vi "Log.vi"(9 "data":variant, 10 "message":string, 11 "level":T1) -> ()   [LabVIEW 2018, in "Logging.lvlib" / "Registry.lvlib"]
uses:
  Registry.lvlib
  Log Levels.ctl
  Log Action Data.ctl
  Registry Actions.ctl
  Logging.lvlib
  Utilities/Utilities.lvlib
panel:
  # "Connector Pane"
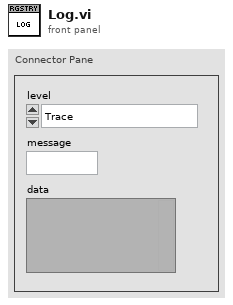
[diagram p1: front panel]
types:
  T1 = typedef "Logging.lvlib/Log Levels.ctl" = enum16{"Trace", "Debug", "Info", "Warning", "Error", "Critical"}
  T2 = typedef "Logging.lvlib/Registry.lvlib/Registry Actions.ctl" = enum16{"Register", "Log", "Enable", "Enable All", "Disable", "Disable All", "List", "Unregister", "Unregister All"}
  T3 = typedef "Logging.lvlib/Registry.lvlib/Log Action Data.ctl" = cluster{"level":T1, "message":string, "data":variant}
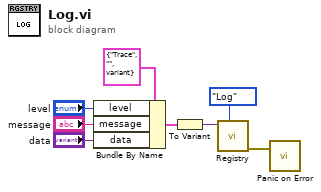
[diagram p0: block diagram]
diagram:
  n1 = Bundle By Name(cluster=T3 {"level"=enum."Trace", "message"="", "data"=variant}, "level"="level", "message"="message", "data"="data") -> (w6:T3)
  n2 = To Variant(anything=w6) -> (Variant=w7:variant)
  n3 = call "Registry.vi"("action"=Registry_Actions."Log", "data in"=w7) -> ("error out"=w1:errorcluster)  [unwired: 8 in, 1 out]
  n4 = call "Panic on Error.vi"("error in (no error)"=w1) -> ()  [unwired: 3 in]
